vi "DUmmy Array.vi"() -> (4 "output array":dbl[](array[numeric]))   [LabVIEW 2013]
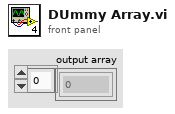
[diagram p1: front panel]
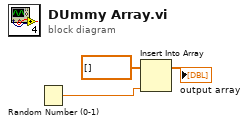
[diagram p0: block diagram]
diagram:
  n1 = Random Number (0-1)() -> (number: 0 to 1=w3:dbl)
  n2 = Insert Into Array(array=dbl[] [], new element=w3) -> (→"output array":dbl[])  [unwired: 1 in]
